vi "Read configuration.vi"(8 "error in":errorcluster, 11 "RTResourceUtilitzation editor node in":refnum<class "RTResourceUtilitzation editor node.lvclass">) -> (0 "error out":errorcluster, 2 "configuration":refnum<class "NISE_CEF_serializable configuration.lvclass">, 3 "RTResourceUtilitzation editor node out":refnum<class "RTResourceUtilitzation editor node.lvclass">)   [LabVIEW 2014, in "RTResourceUtilitzation editor node.lvclass"]
uses:
  RTResourceUtilitzation editor node.lvclass
  <vilib>/NI/Configuration Framework/serializable configuration/NISE_CEF_serializable configuration.lvclass
  RTResourceUtilitzation editor node.lvclass/RTResourceUtilitzation editor node.ctl
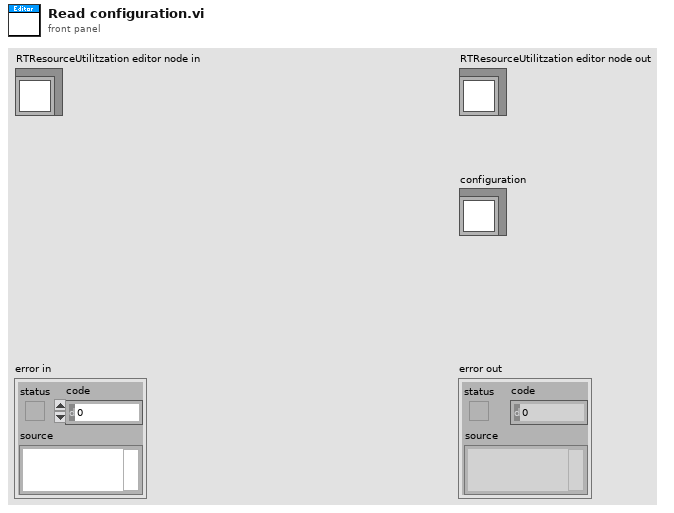
[diagram p1: front panel]
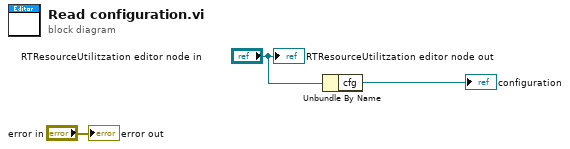
[diagram p0: block diagram]
diagram:
  n1 = Unbundle By Name("RTResourceUtilitzation editor node in") -> ("cfg"=→"configuration":refnum<class "RTResourceUtilitzation configuration.lvclass">)
  "error out" <- "error in"
  "RTResourceUtilitzation editor node out" <- "RTResourceUtilitzation editor node in"
